vi "Convert data.vi"(8 "Error in":errorcluster, 11 "Element in":T3) -> (0 "Error out":errorcluster, 1 "Data out":dbl[][](array[numeric]), 2 "Channels name":string[](array[string]), 3 "Content type":string)   [LabVIEW 2015, in "Logging.lvlib"]
uses:
  Logging.lvlib
  Acquisition/Generic data packet.ctl
  My Graphs/Gps Map Graph coordinates.ctl
  Acquisition/IDRA Data Packet.ctl
  Acquisition/XAM Data Packet.ctl
  Acquisition/Acquisition.lvlib
panel:
  in  "XAM Data Packet":T1
  in  "IDRA Data Packet":T2
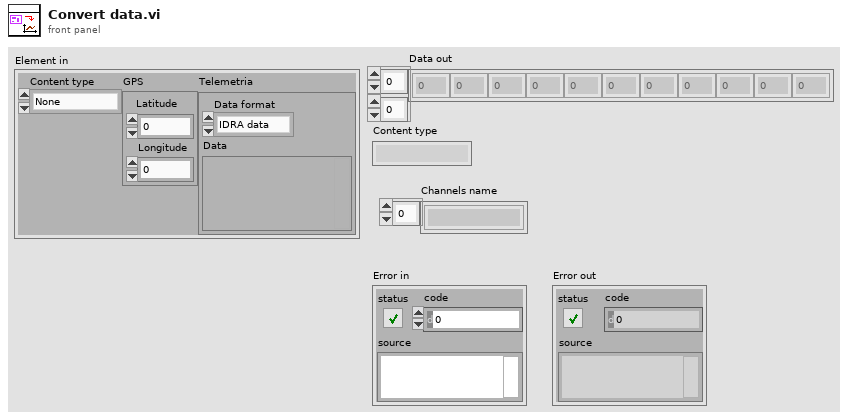
[diagram p1: front panel]
types:
  T1 = typedef "Acquisition.lvlib/XAM Data Packet.ctl" = cluster{"Minutes":u16, "Seconds/100":u16, "Supercap Voltage":sgl, "Battery Voltage":sgl, "Supercap Current":sgl, "Speed":sgl, "EM Temperature":sgl, "ECU Temperature":sgl, "ICE Temperature":sgl, "RPM EM":u16, "RPM ICE":u16, "Cruise Control":bool, "Emergency":bool}
  T2 = typedef "Acquisition.lvlib/IDRA Data Packet.ctl" = cluster{"Minutes":u16, "Seconds/100":u16, "Voltage":sgl, "Current":sgl, "Speed":sgl, "Temperature 1":sgl, "Temperature 2":sgl, "Temperature 3":sgl, "Humidity 1":sgl, "Humidity 2":sgl, "Strategy":u8, "Electric Motor":bool, "Electronics":bool, "Emergency":bool}
  T3 = typedef "Acquisition.lvlib/Generic data packet.ctl" = cluster{"Content type":enum16{"None", "Telemetria", "GPS"}, "GPS":T4, "Telemetria":cluster{"Data format":enum16{"IDRA data", "XAM data"}, "Data":variant}}
  T4 = typedef "Gps Map Graph coordinates.ctl" = cluster{"Latitude":dbl, "Longitude":dbl}
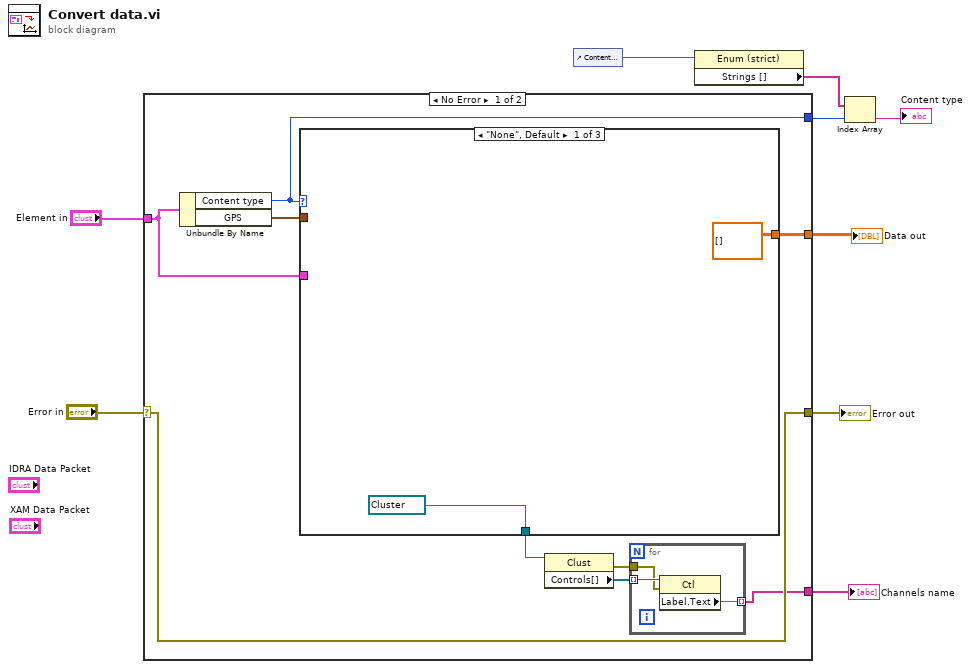
[diagram p0: block diagram]
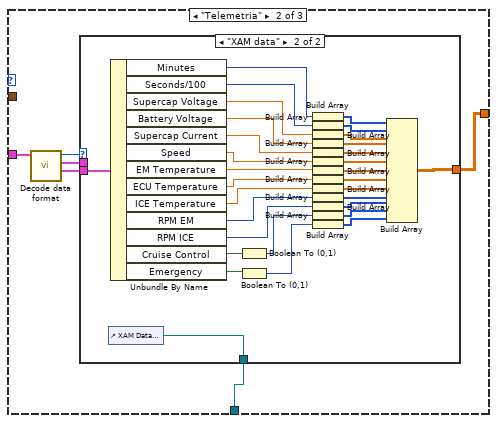
[diagram p2: hidden frame]
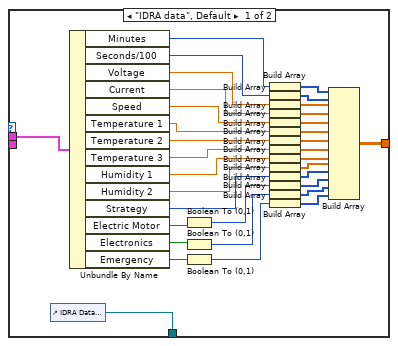
[diagram p3: hidden frame]
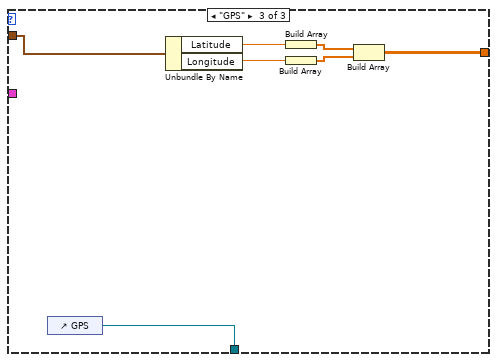
[diagram p4: hidden frame]
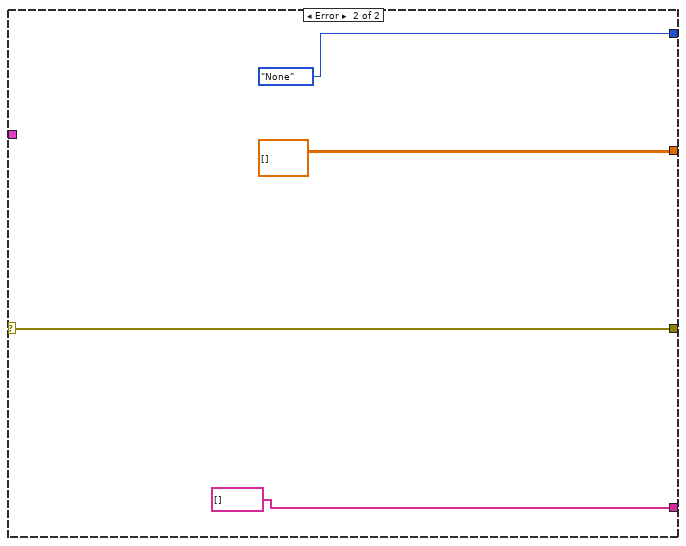
[diagram p5: hidden frame]
diagram:
  n1 = case shown="No Error" "Error in" {
    selector: "Error in" -> [w18 w105]
    tunnel: [w18 w105] -> w8
    tunnel: "Element in" -> [w12 _]
    tunnel: [w17 enum16{"None", "Telemetria", "GPS"}."None" ("Content type")] -> w6
    tunnel: [w16 dbl[][] []] -> w3
    tunnel: [w15 string[] []] -> w7
    frame No Error {
      n2 = Unbundle By Name(w12) -> ("Content type"=w17:enum16{"None", "Telemetria", "GPS"}, "GPS"=w11:T4)
      n3 = case shown="\"None\", Default" w17 {
        tunnel: w11 -> [_ _ w101]
        tunnel: [dbl[][] [] w29 w96] -> w16
        tunnel: [refnum<vi> refnum ("GPS") w26 w95] -> w13
        tunnel: w12 -> [_ w27 _]
        frame "None", Default {
        }
        frame "Telemetria" {
          n4 = call "Decode data format.vi"("Generic packet"=w27) -> ("XAM Data Packet"=w25:T1, "IDRA Data Packet"=w28:T2, "Telemetria.Data format"=w24:enum16{"IDRA data", "XAM data"})  [unwired: 8 in]
          n5 = case shown="\"XAM data\"" w24 {
            tunnel: [w63 w90] -> w29
            tunnel: w28 -> [w31 _]
            tunnel: [w30 w94] -> w26
            tunnel: w25 -> [_ w93]
            frame "IDRA data", Default {
              n6 = control-ref of="IDRA Data Packet"() -> (w30:refnum<vi>)
              n7 = Unbundle By Name(w31) -> ("Minutes"=w46:u16, "Seconds/100"=w62:u16, "Voltage"=w61:sgl, "Current"=w60:sgl, "Speed"=w59:sgl, "Temperature 1"=w58:sgl, "Temperature 2"=w57:sgl, "Temperature 3"=w56:sgl, "Humidity 1"=w55:sgl, "Humidity 2"=w54:sgl, "Strategy"=w53:u8, "Electric Motor"=w52:bool, "Electronics"=w50:bool, "Emergency"=w49:bool)
              n8 = Boolean To (0,1)(Boolean=w52) -> (0, 1=w51:i16)
              n9 = Boolean To (0,1)(Boolean=w50) -> (0, 1=w48:i16)
              n10 = Boolean To (0,1)(Boolean=w49) -> (0, 1=w47:i16)
              n11 = Build Array(w46) -> (w45:u16[])
              n12 = Build Array(w62) -> (w44:u16[])
              n13 = Build Array(w61) -> (w43:sgl[])
              n14 = Build Array(w60) -> (w42:sgl[])
              n15 = Build Array(w59) -> (w41:sgl[])
              n16 = Build Array(w58) -> (w40:sgl[])
              n17 = Build Array(w57) -> (w39:sgl[])
              n18 = Build Array(w56) -> (w38:sgl[])
              n19 = Build Array(w55) -> (w37:sgl[])
              n20 = Build Array(w54) -> (w36:sgl[])
              n21 = Build Array(w53) -> (w35:u8[])
              n22 = Build Array(w51) -> (w34:i16[])
              n23 = Build Array(w48) -> (w33:i16[])
              n24 = Build Array(w47) -> (w32:i16[])
              n25 = Build Array(w45, w44, w43, w42, w41, w40, w39, w38, w37, w36, w35, w34, w33, w32) -> (w63:sgl[][])
            }
            frame "XAM data" {
              n26 = control-ref of="XAM Data Packet"() -> (w94:refnum<vi>)
              n27 = Unbundle By Name(w93) -> ("Minutes"=w88:u16, "Seconds/100"=w85:u16, "Supercap Voltage"=w84:sgl, "Battery Voltage"=w83:sgl, "Supercap Current"=w82:sgl, "Speed"=w81:sgl, "EM Temperature"=w80:sgl, "ECU Temperature"=w79:sgl, "ICE Temperature"=w78:sgl, "RPM EM"=w77:u16, "RPM ICE"=w76:u16, "Cruise Control"=w91:bool, "Emergency"=w92:bool)
              n28 = Boolean To (0,1)(Boolean=w91) -> (0, 1=w75:i16)
              n29 = Boolean To (0,1)(Boolean=w92) -> (0, 1=w74:i16)
              n30 = Build Array(w88) -> (w89:u16[])
              n31 = Build Array(w85) -> (w87:u16[])
              n32 = Build Array(w84) -> (w86:sgl[])
              n33 = Build Array(w83) -> (w73:sgl[])
              n34 = Build Array(w82) -> (w72:sgl[])
              n35 = Build Array(w81) -> (w64:sgl[])
              n36 = Build Array(w80) -> (w65:sgl[])
              n37 = Build Array(w79) -> (w66:sgl[])
              n38 = Build Array(w78) -> (w67:sgl[])
              n39 = Build Array(w77) -> (w68:u16[])
              n40 = Build Array(w76) -> (w69:u16[])
              n41 = Build Array(w75) -> (w70:i16[])
              n42 = Build Array(w74) -> (w71:i16[])
              n43 = Build Array(w89, w87, w86, w73, w72, w64, w65, w66, w67, w68, w69, w70, w71) -> (w90:sgl[][])
            }
          }
        }
        frame "GPS" {
          n44 = control-ref of="GPS"() -> (w95:refnum<vi>)
          n45 = Unbundle By Name(w101) -> ("Latitude"=w97:dbl, "Longitude"=w98:dbl)
          n46 = Build Array(w97) -> (w100:dbl[])
          n47 = Build Array(w98) -> (w99:dbl[])
          n48 = Build Array(w100, w99) -> (w96:dbl[][])
        }
      }
      n49 = property class="Clust"(reference=w13) -> (error out=w10:errorcluster, "Controls[]"=w14:refnum<vi>[])  [unwired: 1 in, 1 out]
      n50 = for {
        tunnel: [w21] -> w15 mode=indexing
        tunnel: w14 -> [w20] mode=indexing
        tunnel: w10 -> [w19]
        n51 = property class="Ctl"(reference=w20, error in=w19) -> ("Label.Text"=w21:string)  [unwired: 2 out]
      }
    }
    frame Error {
    }
  }
  "Error out" <- w8
  "Data out" <- w3
  "Channels name" <- w7
  n52 = control-ref of="Content type"() -> (w1:refnum<vi>)
  n53 = property class="Enum (strict)"(reference=w1) -> ("Strings []"=w5:string[])  [unwired: 1 in, 2 out]
  n54 = Index Array(array=w5, index=w6) -> (element=→"Content type":string)
